vi "point_in_irons_or_dead_downwind.vi"(10 "NotifierReff":T1, 11 "Point":T2 {"North" format="%#_10f"; "East" format="%#_8f"}) -> (1 "Dead downwind?":bool, 2 "In irons?":bool, 3 "In irons or dead downwind?":bool)   [LabVIEW 2013]
doc: "Checks if next waypoint will require sailing upwind into irons or going dead downwind."
uses:
  Data/TypeDefs/UTM Location.ctl
  Data/TypeDefs/Notifiers.ctl
  Data/TypeDefs/Sail Set Suggestions.ctl
  Data/TypeDefs/Rudder Set Suggestions.ctl
  Data/TypeDefs/OverrideInformation.ctl
  Data/TypeDefs/OverrideMode.ctl
  Data/TypeDefs/MotorSetup.ctl
  Data/TypeDefs/DynamixelSetupInfo.ctl
  Data/TypeDefs/AirmarStatus.ctl
  Data/TypeDefs/HardwareOnline.ctl
  Data/TypeDefs/DynamixelCycleTracker.ctl
  Data/TypeDefs/RC Input Values.ctl
  Logic/Classes/Waypoint/Waypoint.lvclass
  Angles/Angle/Angle.lvclass
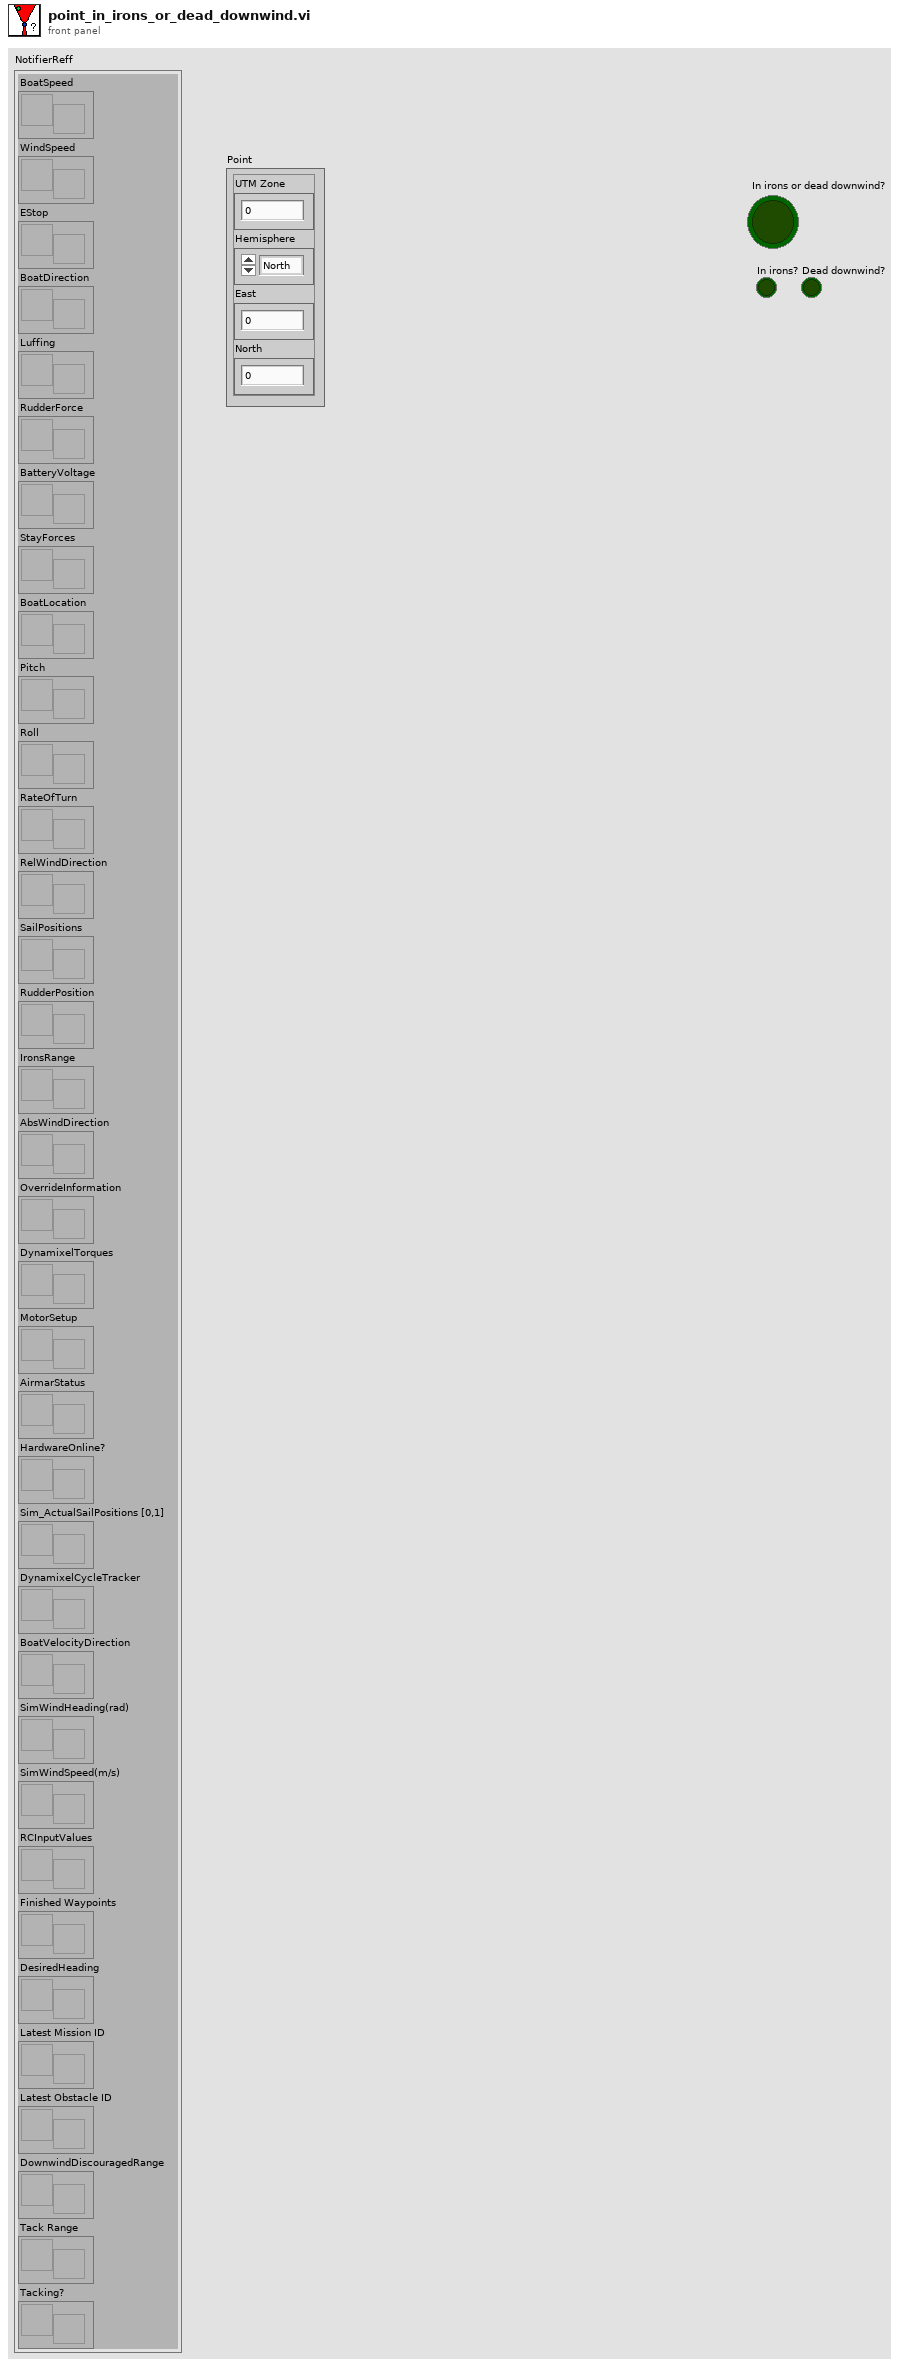
[diagram p1: front panel]
types:
  T1 = typedef "Notifiers.ctl" = cluster{"BoatSpeed":refnum<notifier>, "WindSpeed":refnum<notifier>, "EStop":refnum<notifier>, "BoatDirection":refnum<notifier>, "Luffing":refnum<notifier>, "RudderForce":refnum<notifier>, "BatteryVoltage":refnum<notifier>, "StayForces":refnum<notifier>, "BoatLocation":refnum<notifier>, "Pitch":refnum<notifier>, "Roll":refnum<notifier>, "RateOfTurn":refnum<notifier>, "RelWindDirection":refnum<notifier>, "SailPositions":refnum<notifier>, "RudderPosition":refnum<notifier>, "IronsRange":refnum<notifier>, "AbsWindDirection":refnum<notifier>, "OverrideInformation":refnum<notifier>, "DynamixelTorques":refnum<notifier>, "MotorSetup":refnum<notifier>, "AirmarStatus":refnum<notifier>, "HardwareOnline?":refnum<notifier>, "Sim_ActualSailPositions [0,1]":refnum<notifier>, "DynamixelCycleTracker":refnum<notifier>, "BoatVelocityDirection":refnum<notifier>, "SimWindHeading(rad)":refnum<notifier>, "SimWindSpeed(m/s)":refnum<notifier>, "RCInputValues":refnum<notifier>, "Finished Waypoints":refnum<notifier>, "DesiredHeading":refnum<notifier>, "Latest Mission ID":refnum<notifier>, "Latest Obstacle ID":refnum<notifier>, "DownwindDiscouragedRange":refnum<notifier>, "Tack Range":refnum<notifier>, "Tacking?":refnum<notifier>}
  T2 = typedef "UTM Location.ctl" = cluster{"UTM Zone":dbl, "Hemisphere":enum16{"North", "South"}, "East":dbl, "North":dbl}
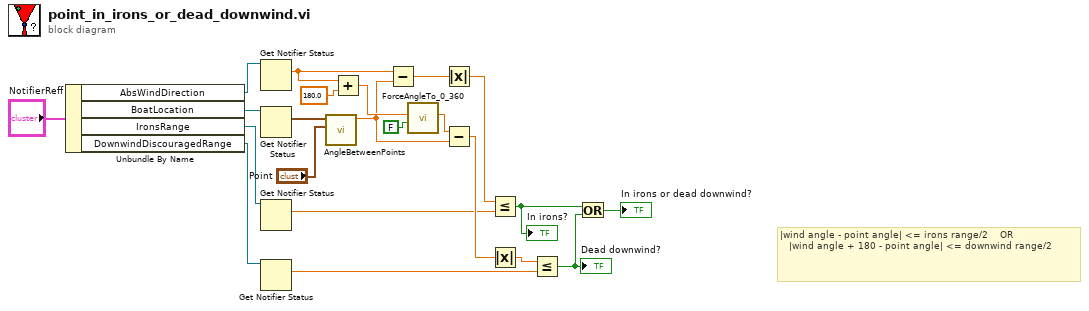
[diagram p0: block diagram]
diagram:
  # "|wind angle - point angle| <= irons range/2    OR\n   |wind angle + 180 - point angle| <= downwind range/2"
  n1 = Unbundle By Name("NotifierReff") -> ("AbsWindDirection"=w6:refnum<notifier>, "BoatLocation"=w9:refnum<notifier>, "IronsRange"=w8:refnum<notifier>, "DownwindDiscouragedRange"=w2:refnum<notifier>)
  n2 = Get Notifier Status(notifier=w6) -> (current notification=w5:dbl)  [unwired: 1 in, 4 out]
  n3 = Get Notifier Status(notifier=w9) -> (current notification=w4:T2)  [unwired: 1 in, 4 out]
  n4 = Get Notifier Status(notifier=w8) -> (current notification=w3:dbl)  [unwired: 1 in, 4 out]
  n5 = Get Notifier Status(notifier=w2) -> (current notification=w1:dbl)  [unwired: 1 in, 4 out]
  n6 = call "AngleBetweenPoints.vi"("Point 2"="Point", "Point 1"=w4) -> ("Angle from P1 to P2"=w15:dbl)  [unwired: 9 in]
  n7 = Add(x=w5, y=180.0) -> (x+y=w17:dbl)
  n8 = Subtract(x=w5, y=w15) -> (x-y=w22:dbl)
  n9 = call "ForceAngleTo_0_360.vi"("Use angle class? (T)"=FALSE, "Angle in"=w17) -> ("Forced Angle"=w16:dbl)  [unwired: 7 in, 2 out]
  n10 = Absolute Value(x=w22) -> (abs(x)=w21:dbl)
  n11 = Subtract(x=w16, y=w15) -> (x-y=w13:dbl)
  n12 = Less Or Equal?(x=w21, y=w3) -> (x <= y?=w12:bool)
  "In irons?" <- w12
  n13 = Absolute Value(x=w13) -> (abs(x)=w14:dbl)
  n14 = Less Or Equal?(x=w14, y=w1) -> (x <= y?=w10:bool)
  "Dead downwind?" <- w10
  n15 = Or(x=w12, y=w10) -> (x .or. y?=→"In irons or dead downwind?":bool)
